vi "Master.vi"() -> ()   [LabVIEW 2017]
uses:
  Globle/Trigger Home Screen.vi
panel:
  in  "Master\nBreakdown\nDetail":bool
  out "appended array":refnum<vi>[](array[refnum])
  in  "Cancel Button - Archive":bool
  in  "Reason":bool
  in  "Escallation":bool
  in  "Shift":bool
  in  "User":bool
  # "MASTER"
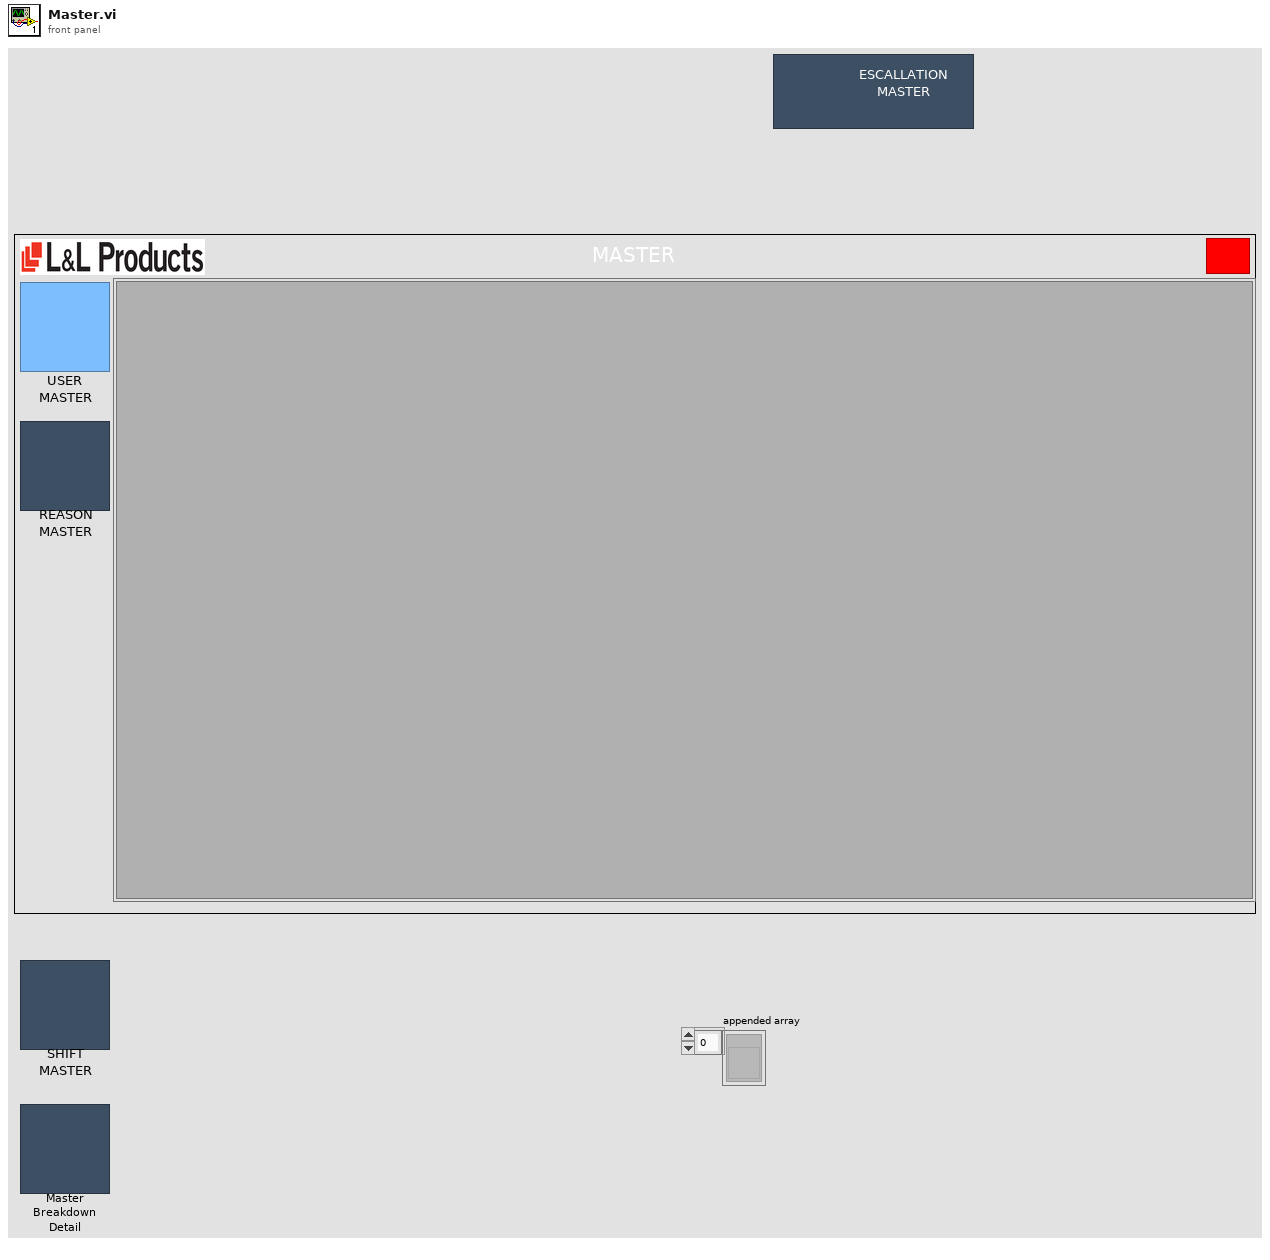
[diagram p1: front panel]
types:
  T1 = enum32{"invalid app kind", "Development System", "Run Time System", "Student Edition", "Embedded LabVIEW", "Evaluation", "Custom"}
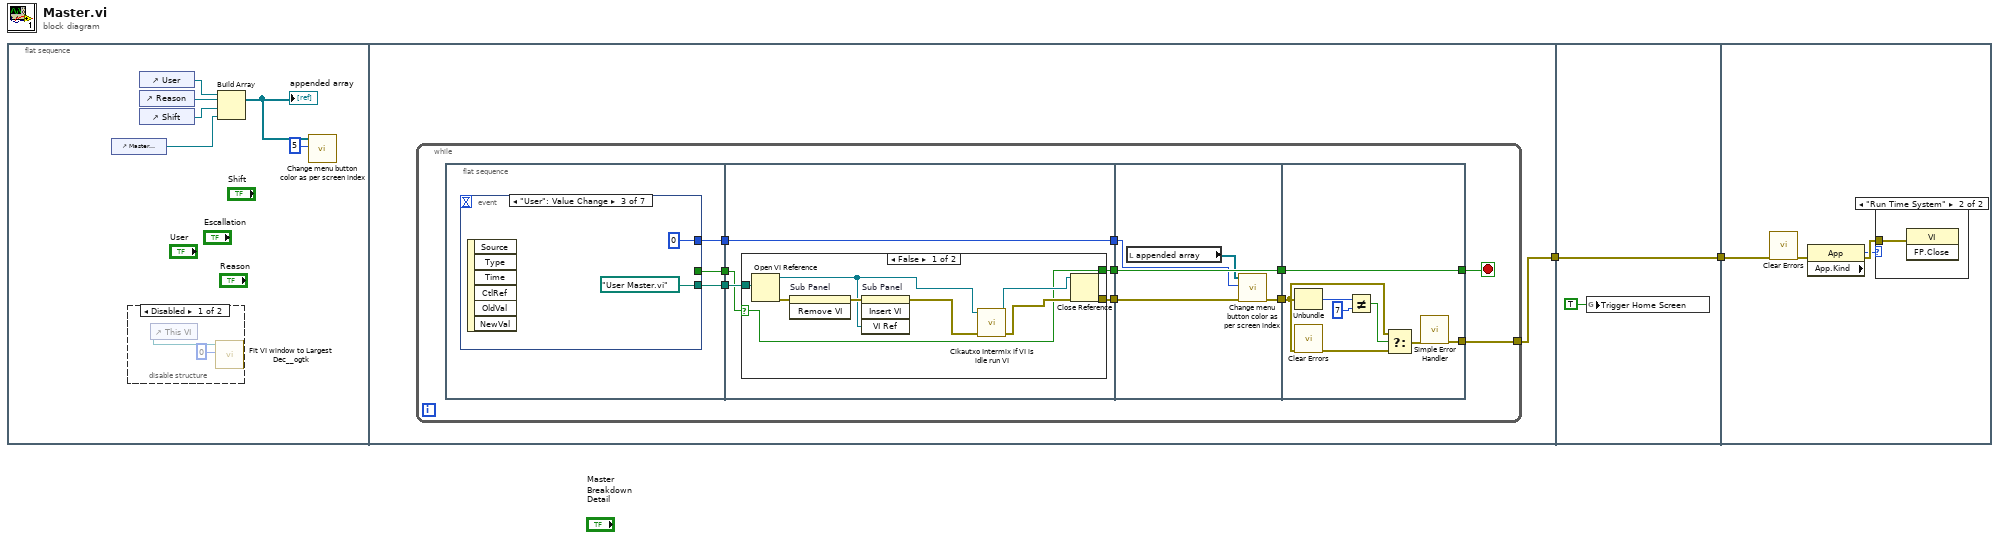
[diagram p0: block diagram]
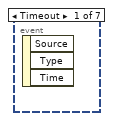
[diagram p3: hidden frame]
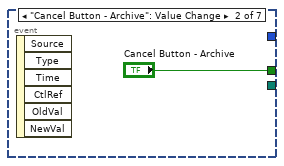
[diagram p4: hidden frame]
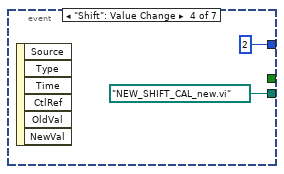
[diagram p5: hidden frame]
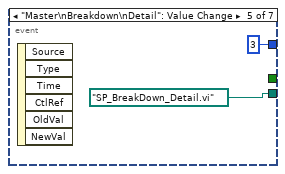
[diagram p6: hidden frame]
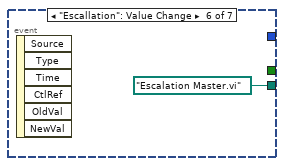
[diagram p7: hidden frame]
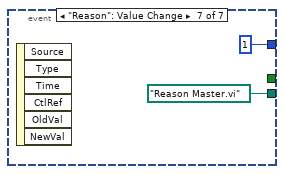
[diagram p8: hidden frame]
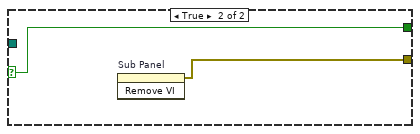
[diagram p9: hidden frame]
diagram:
  n1 = flat-sequence {
    tunnel: [w11] -> w2
    tunnel: w2 -> [w65]
    tunnel: [w65] -> w1
    tunnel: w1 -> [w69]
    frame #0 {
      n2 = control-ref of="Master\nBreakdown\nDetail"() -> (w3:refnum<vi>)
      n3 = disable-structure shown="Disabled" {
        frame Disabled {
          n4 = control-ref of="This VI"() -> (w10:refnum<vi>)
          n5 = call <userlib>:"Fit VI window to Largest Dec__ogtk.vi"("border spacing (2 px)"=0, "VI Ref (calling VI)"=w10) -> ()  [unwired: 4 in, 2 out]
        }
        frame Enabled {
        }
      }
      n6 = control-ref of="User"() -> (w8:refnum<vi>)
      n7 = control-ref of="Reason"() -> (w7:refnum<vi>)
      n8 = control-ref of="Shift"() -> (w6:refnum<vi>)
      n9 = Build Array(w8, w7, w6, w3) -> (w5:refnum<vi>[])
      "appended array" <- w5
      n10 = call "Change menu button color as per screen index.vi"("Screen Index"=5, "Array"=w5) -> ()  [unwired: 9 in, 1 out]
    }
    frame #1 {
      n11 = while {
        tunnel: [w18] -> w11
        stop <- w21 stop-if-true
        n12 = flat-sequence {
          tunnel: [w24] -> w20
          tunnel: [w23] -> w19
          tunnel: [w22] -> w12
          tunnel: w20 -> [w36]
          tunnel: w19 -> [w38]
          tunnel: [w35] -> w17
          tunnel: [w39] -> w15
          tunnel: [w37] -> w13
          tunnel: w12 -> [w37]
          tunnel: w17 -> [w55]
          tunnel: [w55] -> w16
          tunnel: w15 -> [w52]
          tunnel: [w51] -> w14
          tunnel: w13 -> [w53]
          tunnel: [w63] -> w21
          tunnel: w16 -> [w63]
          tunnel: w14 -> [w56]
          tunnel: [w57] -> w18
          frame #0 {
            n13 = event shown="[2] \"User\": Value Change" {
              selector: _ -> [_ _ _ _ _ _ _]
              dyn-events: _ -> [_ _ _ _ _ _ _]
              timeout: _ -> [_ _ _ _ _ _ _]
              tunnel: [_ "Cancel Button - Archive" _ _ _ _ _] -> w24
              tunnel: [_ _ path "User Master.vi" ("vi path") path "NEW_SHIFT_CAL_new.vi" ("vi path") path "SP_BreakDown_Detail.vi" ("vi path") path "Escalation Master.vi" ("vi path") path "Reason Master.vi" ("vi path")] -> w23
              tunnel: [_ _ 0 2 3 _ 1] -> w22
              event Timeout {
                n14 = event-data() -> ()  [unwired: 1 in, 3 out]
              }
              event "Cancel Button - Archive": Value Change {
                n15 = event-data() -> ()  [unwired: 1 in, 6 out]
              }
              event "User": Value Change {
                n16 = event-data() -> ()  [unwired: 1 in, 6 out]
              }
              event "Shift": Value Change {
                n17 = event-data() -> ()  [unwired: 1 in, 6 out]
              }
              event "Master\nBreakdown\nDetail": Value Change {
                n18 = event-data() -> ()  [unwired: 1 in, 6 out]
              }
              event "Escallation": Value Change {
                n19 = event-data() -> ()  [unwired: 1 in, 6 out]
              }
              event "Reason": Value Change {
                n20 = event-data() -> ()  [unwired: 1 in, 6 out]
              }
            }
          }
          frame #1 {
            n21 = case shown="False" w36 {
              selector: w36 -> [w40 w49]
              tunnel: [w48 w50] -> w39
              tunnel: w38 -> [w46 _]
              tunnel: [w40 w49] -> w35
              frame False {
                n22 = Open VI Reference(vi path=w46) -> (vi reference=w42:refnum<vi>, error out=w45:errorcluster)  [unwired: 5 in]
                n23 = invoke on="Sub Panel" class="SubPnl" method="Remove VI"(error in=w45) -> (error out=w47:errorcluster)  [unwired: 2 in, 2 out]
                n24 = invoke on="Sub Panel" class="SubPnl" method="Insert VI"(error in=w47, "VI Ref"=w42) -> (error out=w44:errorcluster)  [unwired: 2 in, 3 out]
                n25 = call "Cikautxo Intermix if VI is idle run VI.vi"("error in (no error)"=w44, "VI in"=w42) -> ("error out"=w43:errorcluster, "VI out"=w41:refnum<vi>)  [unwired: 8 in]
                n26 = Close Reference(reference=w41, error in (no error)=w43) -> (error out=w48:errorcluster)
              }
              frame True {
                n27 = invoke on="Sub Panel" class="SubPnl" method="Remove VI"() -> (error out=w50:errorcluster)  [unwired: 3 in, 2 out]
              }
            }
          }
          frame #2 {
            n28 = local read "appended array"() -> (w54:refnum<vi>[])
            n29 = call "Change menu button color as per screen index.vi"("error in (no error)"=w52, "Screen Index"=w53, "Array"=w54) -> ("error out"=w51:errorcluster)  [unwired: 8 in]
          }
          frame #3 {
            n30 = Unbundle(w56) -> ("code"=w62:i32)  [unwired: 2 out]
            n31 = call <vilib>:"Clear Errors.vi"("error in (no error)"=w56) -> ("error out"=w59:errorcluster)  [unwired: 5 in, 1 out]
            n32 = Not Equal?(x=w62, y=7) -> (x != y?=w60:bool)
            n33 = Select(t=w56, s=w60, f=w59) -> (s? t:f=w58:errorcluster)
            n34 = call <vilib>:"Simple Error Handler.vi"("error in (no error)"=w58) -> ("error out"=w57:errorcluster)  [unwired: 4 in, 4 out]
          }
        }
      }
    }
    frame #2 {
      n35 = global write "Trigger Home Screen.vi" "Trigger Home Screen"(TRUE ("Trigger Home Screen")) -> ()
    }
    frame #3 {
      n36 = call <vilib>:"Clear Errors.vi"("error in (no error)"=w69) -> ("error out"=w68:errorcluster)  [unwired: 5 in, 1 out]
      n37 = property class="App"(error in=w68) -> (error out=w67:errorcluster, "App.Kind"=w66:T1)  [unwired: 1 in, 1 out]
      n38 = case shown="\"Run Time System\"" w66 {
        tunnel: w67 -> [_ w70]
        frame "Development System", Default {
        }
        frame "Run Time System" {
          n39 = invoke class="VI" method="FP.Close"(error in=w70) -> ()  [unwired: 2 in, 3 out]
        }
      }
    }
  }
